vi "Min Pixel x1 (SubVI).vi"(10 "Pixel 2":u8, 11 "Pixel 1":u8) -> (3 "Min Pixel":u8)   [LabVIEW 2015]
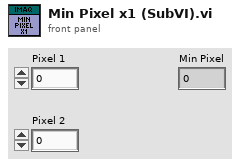
[diagram p1: front panel]
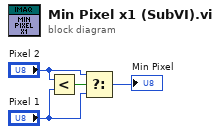
[diagram p0: block diagram]
diagram:
  n1 = Less?(x="Pixel 2", y="Pixel 1") -> (x < y?=w2:bool)
  n2 = Select(t="Pixel 2", s=w2, f="Pixel 1") -> (s? t:f=→"Min Pixel":u8)
